vi "RS_table.vi"(1 "RSpoints":T1[](array[typedef])) -> (0 "Table":string[][](array[string]))   [LabVIEW 2016]
uses:
  StressCalculations/point_data.ctl
  Report/report_mods.ctl
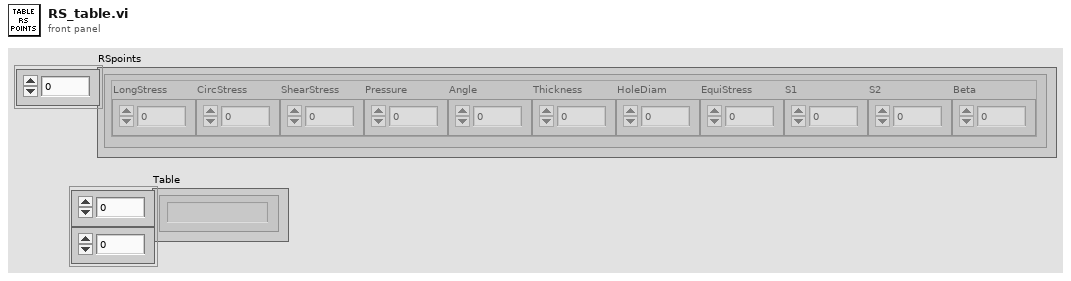
[diagram p1: front panel]
types:
  T1 = typedef "point_data.ctl" = cluster{"LongStress":dbl, "CircStress":dbl, "ShearStress":dbl, "Pressure":dbl, "Angle":dbl, "Thickness":dbl, "HoleDiam":dbl, "EquiStress":dbl, "S1":dbl, "S2":dbl, "Beta":dbl}
  T2 = typedef "report_mods.ctl" = enum16{"Init", "Table", "Graph", "TablefromGraph", "End"}
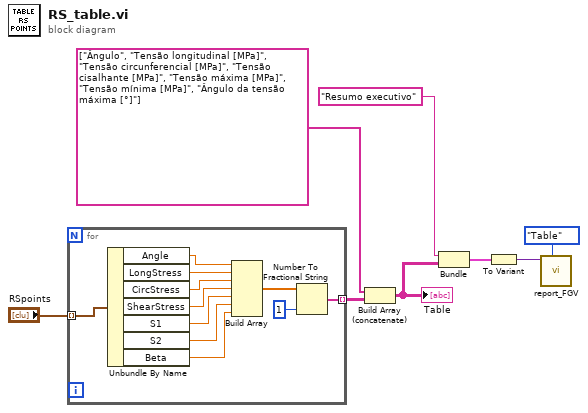
[diagram p0: block diagram]
diagram:
  n1 = for {
    tunnel: "RSpoints" -> [w19] mode=indexing
    tunnel: [w12] -> w7 mode=indexing
    n2 = Unbundle By Name(w19) -> ("Angle"=w18:dbl, "LongStress"=w17:dbl, "CircStress"=w16:dbl, "ShearStress"=w15:dbl, "S1"=w11:dbl, "S2"=w10:dbl, "Beta"=w9:dbl)
    n3 = Build Array(w18, w17, w16, w15, w11, w10, w9) -> (w14:dbl[])
    n4 = Number To Fractional String(number=w14, precision (6)=i16 1) -> (F-format string=w12:string[])  [unwired: 2 in]
  }
  n5 = Build Array (concatenate)(string[] ["Ângulo", "Tensão longitudinal [MPa]", "Tensão circunferencial [MPa]", "Tensão cisalhante [MPa]", "Tensão máxima [MPa]", "Tensão mínima [MPa]", "Ângulo da tensão máxima [°]"] ("element"), w7) -> (w5:string[][])
  "Table" <- w5
  n6 = Bundle("ShearStress"="Resumo executivo", w5) -> (w4:cluster{"ShearStress":string, string[][]})  [unwired: 1 in]
  n7 = To Variant(anything=w4) -> (Variant=w3:variant)
  n8 = call "report_FGV.vi"("report_mods"=report_mods."Table", "Data in"=w3) -> ()  [unwired: 9 in, 1 out]
